vi "In_Range(SubVI).vi"(9 "Proccess Variable":dbl, 10 "AC estimate (Vrms)":dbl, 11 "Setpoint":dbl) -> (1 "In Range?":bool, 3 "coerced(x)":dbl)   [LabVIEW 2019]
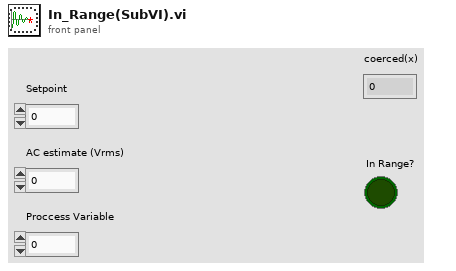
[diagram p1: front panel]
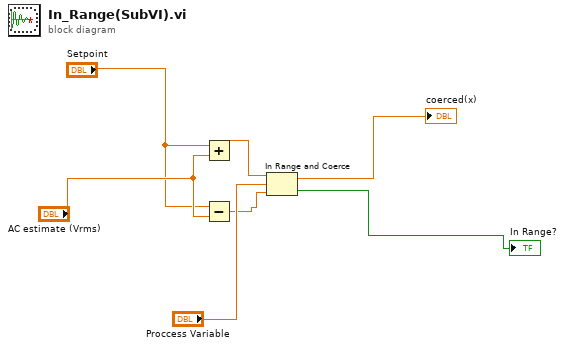
[diagram p0: block diagram]
diagram:
  n1 = Add(x="Setpoint", y="AC estimate (Vrms)") -> (x+y=w4:dbl)
  n2 = Subtract(x="Setpoint", y="AC estimate (Vrms)") -> (x-y=w3:dbl)
  n3 = In Range and Coerce(upper limit=w4, x="Proccess Variable", lower limit=w3) -> (coerced(x)=→"coerced(x)":dbl, In Range?=→"In Range?":bool)
